vi "TrajectoryBegin.vi"(8 "error in (no error)":errorcluster) -> (0 "error out":errorcluster)   [LabVIEW 2023]
uses:
  TrajectoryGlobals.vi
  <vilib>/Rock Robotics/WPI/ThirdParty/JAS_Junk/TrajLib/Trajectory_Library.lvlib
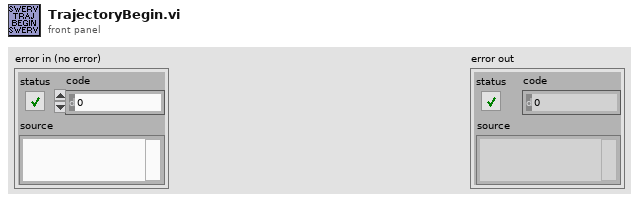
[diagram p1: front panel]
types:
  T1 = typedef "Trajectory_Library.lvlib/TRAJECTORY.ctl" = cluster{"TotalTImeSecs":dbl, "States":T2[]}
  T2 = typedef "Trajectory_Library.lvlib/TRAJ_STATE.ctl" = cluster{"TimeSeconds":dbl, "Velocity":dbl, "Acceleration":dbl, "POSE":T3, "Curvature":dbl}
  T3 = typedef "Trajectory_Library.lvlib/POSE2D.ctl" = cluster{"TRANSLATION":T4, "ROTATION":T5}
  T4 = typedef "Trajectory_Library.lvlib/TRANSLATION2D.ctl" = cluster{"X":dbl, "Y":dbl}
  T5 = typedef "Trajectory_Library.lvlib/ROTATION2D.ctl" = cluster{"VALUE":dbl, "COS":dbl, "SIN":dbl}
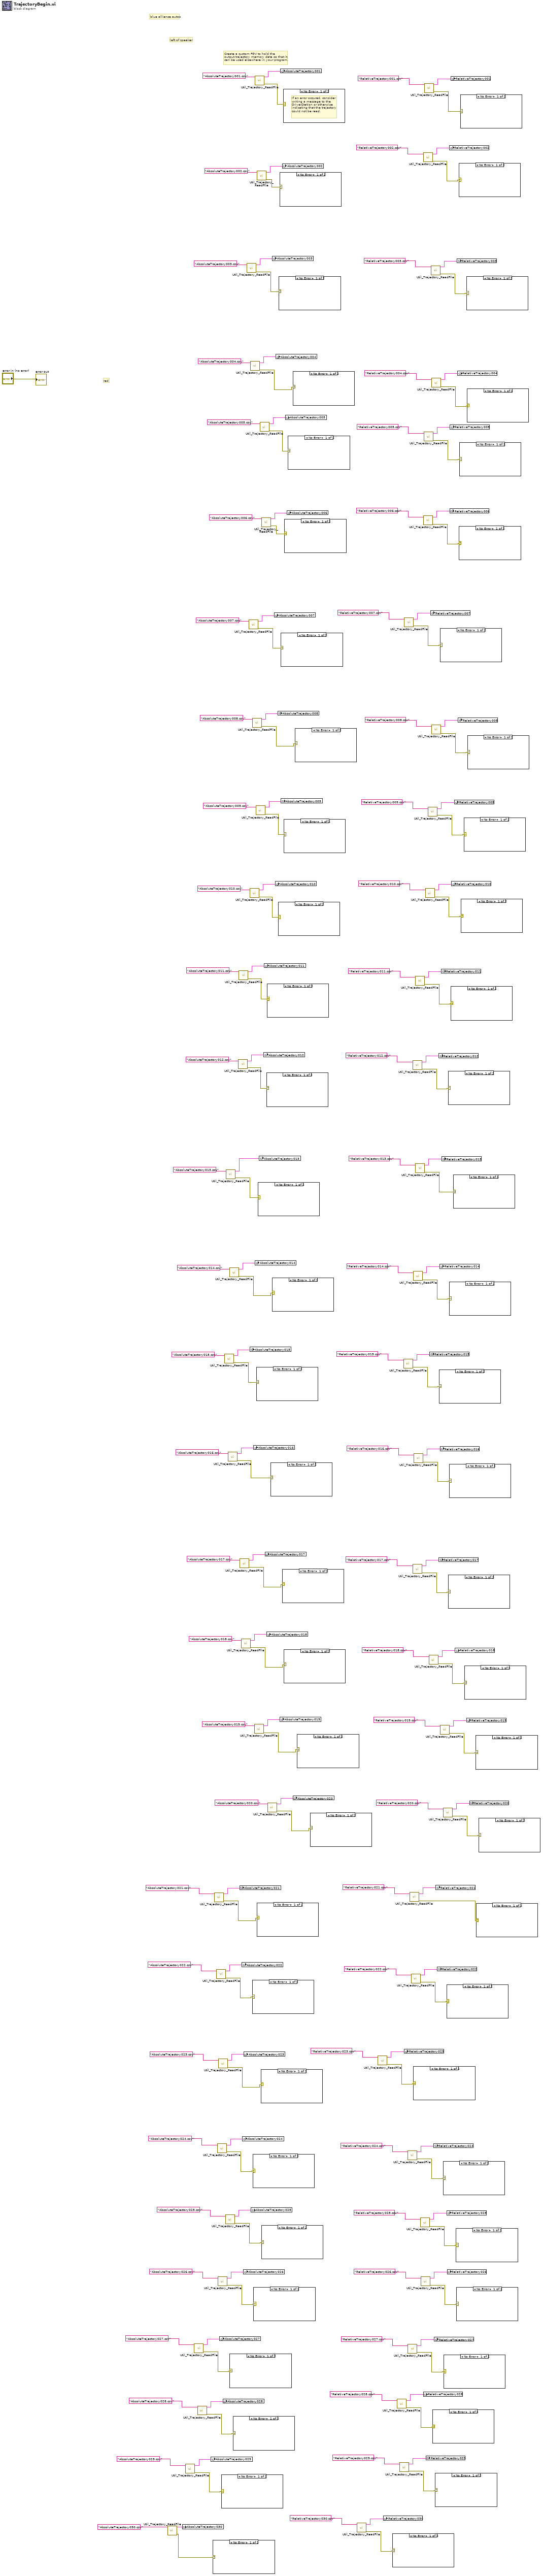
[diagram p0: block diagram]
diagram:
  # "red"
  # "Create a custom FGV to hold the \noutput trajectory memory data so that it\ncan be used elsewhere in your program."
  # "left of speaker"
  # "blue allience autos"
  n1 = call <vilib>:"Util_Trajectory_ReadFile.vi"("FileName"="AbsoluteTrajectory030.csv") -> ("error out"=w91:errorcluster, "outTRAJECTORY"=w92:T1)  [unwired: 8 in, 1 out]
  n2 = global write "TrajectoryGlobals.vi" "AbsoluteTrajectory030"(w92) -> ()
  n3 = call <vilib>:"Util_Trajectory_ReadFile.vi"("FileName"="AbsoluteTrajectory029.csv") -> ("error out"=w94:errorcluster, "outTRAJECTORY"=w95:T1)  [unwired: 8 in, 1 out]
  n4 = call <vilib>:"Util_Trajectory_ReadFile.vi"("FileName"="AbsoluteTrajectory027.csv") -> ("error out"=w100:errorcluster, "outTRAJECTORY"=w101:T1)  [unwired: 8 in, 1 out]
  n5 = call <vilib>:"Util_Trajectory_ReadFile.vi"("FileName"="AbsoluteTrajectory028.csv") -> ("error out"=w97:errorcluster, "outTRAJECTORY"=w98:T1)  [unwired: 8 in, 1 out]
  n6 = global write "TrajectoryGlobals.vi" "AbsoluteTrajectory029"(w95) -> ()
  n7 = case shown="No Error" w91 {
    frame No Error {
    }
    frame Error {
    }
  }
  n8 = call <vilib>:"Util_Trajectory_ReadFile.vi"("FileName"="AbsoluteTrajectory021.csv") -> ("error out"=w118:errorcluster, "outTRAJECTORY"=w119:T1)  [unwired: 8 in, 1 out]
  n9 = call <vilib>:"Util_Trajectory_ReadFile.vi"("FileName"="AbsoluteTrajectory022.csv") -> ("error out"=w115:errorcluster, "outTRAJECTORY"=w116:T1)  [unwired: 8 in, 1 out]
  n10 = call <vilib>:"Util_Trajectory_ReadFile.vi"("FileName"="AbsoluteTrajectory024.csv") -> ("error out"=w109:errorcluster, "outTRAJECTORY"=w110:T1)  [unwired: 8 in, 1 out]
  n11 = call <vilib>:"Util_Trajectory_ReadFile.vi"("FileName"="AbsoluteTrajectory026.csv") -> ("error out"=w103:errorcluster, "outTRAJECTORY"=w104:T1)  [unwired: 8 in, 1 out]
  n12 = call <vilib>:"Util_Trajectory_ReadFile.vi"("FileName"="AbsoluteTrajectory023.csv") -> ("error out"=w112:errorcluster, "outTRAJECTORY"=w113:T1)  [unwired: 8 in, 1 out]
  n13 = global write "TrajectoryGlobals.vi" "AbsoluteTrajectory027"(w101) -> ()
  n14 = case shown="No Error" w94 {
    frame No Error {
    }
    frame Error {
    }
  }
  n15 = global write "TrajectoryGlobals.vi" "AbsoluteTrajectory028"(w98) -> ()
  n16 = call <vilib>:"Util_Trajectory_ReadFile.vi"("FileName"="AbsoluteTrajectory015.csv") -> ("error out"=w142:errorcluster, "outTRAJECTORY"=w143:T1)  [unwired: 8 in, 1 out]
  n17 = call <vilib>:"Util_Trajectory_ReadFile.vi"("FileName"="AbsoluteTrajectory025.csv") -> ("error out"=w106:errorcluster, "outTRAJECTORY"=w107:T1)  [unwired: 8 in, 1 out]
  n18 = call <vilib>:"Util_Trajectory_ReadFile.vi"("FileName"="AbsoluteTrajectory013.csv") -> ("error out"=w136:errorcluster, "outTRAJECTORY"=w137:T1)  [unwired: 8 in, 1 out]
  n19 = call <vilib>:"Util_Trajectory_ReadFile.vi"("FileName"="AbsoluteTrajectory016.csv") -> ("error out"=w139:errorcluster, "outTRAJECTORY"=w140:T1)  [unwired: 8 in, 1 out]
  n20 = call <vilib>:"Util_Trajectory_ReadFile.vi"("FileName"="AbsoluteTrajectory014.csv") -> ("error out"=w133:errorcluster, "outTRAJECTORY"=w134:T1)  [unwired: 8 in, 1 out]
  n21 = case shown="No Error" w100 {
    frame No Error {
    }
    frame Error {
    }
  }
  n22 = case shown="No Error" w97 {
    frame No Error {
    }
    frame Error {
    }
  }
  n23 = call <vilib>:"Util_Trajectory_ReadFile.vi"("FileName"="AbsoluteTrajectory012.csv") -> ("error out"=w147:errorcluster, "outTRAJECTORY"=w145:T1)  [unwired: 8 in, 1 out]
  n24 = call <vilib>:"Util_Trajectory_ReadFile.vi"("FileName"="AbsoluteTrajectory011.csv") -> ("error out"=w150:errorcluster, "outTRAJECTORY"=w148:T1)  [unwired: 8 in, 1 out]
  n25 = call <vilib>:"Util_Trajectory_ReadFile.vi"("FileName"="AbsoluteTrajectory017.csv") -> ("error out"=w130:errorcluster, "outTRAJECTORY"=w131:T1)  [unwired: 8 in, 1 out]
  n26 = global write "TrajectoryGlobals.vi" "AbsoluteTrajectory021"(w119) -> ()
  n27 = call <vilib>:"Util_Trajectory_ReadFile.vi"("FileName"="AbsoluteTrajectory018.csv") -> ("error out"=w127:errorcluster, "outTRAJECTORY"=w128:T1)  [unwired: 8 in, 1 out]
  n28 = global write "TrajectoryGlobals.vi" "AbsoluteTrajectory022"(w116) -> ()
  n29 = global write "TrajectoryGlobals.vi" "AbsoluteTrajectory024"(w110) -> ()
  n30 = global write "TrajectoryGlobals.vi" "AbsoluteTrajectory026"(w104) -> ()
  n31 = global write "TrajectoryGlobals.vi" "AbsoluteTrajectory023"(w113) -> ()
  n32 = call <vilib>:"Util_Trajectory_ReadFile.vi"("FileName"="AbsoluteTrajectory003.csv") -> ("error out"=w160:errorcluster, "outTRAJECTORY"=w161:T1)  [unwired: 8 in, 1 out]
  n33 = call <vilib>:"Util_Trajectory_ReadFile.vi"("FileName"="AbsoluteTrajectory007.csv") -> ("error out"=w172:errorcluster, "outTRAJECTORY"=w173:T1)  [unwired: 8 in, 1 out]
  n34 = call <vilib>:"Util_Trajectory_ReadFile.vi"("FileName"="AbsoluteTrajectory010.csv") -> ("error out"=w153:errorcluster, "outTRAJECTORY"=w151:T1)  [unwired: 8 in, 1 out]
  n35 = global write "TrajectoryGlobals.vi" "AbsoluteTrajectory015"(w143) -> ()
  n36 = call <vilib>:"Util_Trajectory_ReadFile.vi"("FileName"="AbsoluteTrajectory004.csv") -> ("error out"=w157:errorcluster, "outTRAJECTORY"=w158:T1)  [unwired: 8 in, 1 out]
  n37 = global write "TrajectoryGlobals.vi" "AbsoluteTrajectory025"(w107) -> ()
  n38 = case shown="No Error" w115 {
    frame No Error {
    }
    frame Error {
    }
  }
  n39 = call <vilib>:"Util_Trajectory_ReadFile.vi"("FileName"="AbsoluteTrajectory008.csv") -> ("error out"=w169:errorcluster, "outTRAJECTORY"=w170:T1)  [unwired: 8 in, 1 out]
  n40 = case shown="No Error" w109 {
    frame No Error {
    }
    frame Error {
    }
  }
  n41 = global write "TrajectoryGlobals.vi" "AbsoluteTrajectory016"(w140) -> ()
  n42 = case shown="No Error" w103 {
    frame No Error {
    }
    frame Error {
    }
  }
  n43 = call <vilib>:"Util_Trajectory_ReadFile.vi"("FileName"="AbsoluteTrajectory019.csv") -> ("error out"=w124:errorcluster, "outTRAJECTORY"=w125:T1)  [unwired: 8 in, 1 out]
  n44 = global write "TrajectoryGlobals.vi" "AbsoluteTrajectory014"(w134) -> ()
  n45 = call <vilib>:"Util_Trajectory_ReadFile.vi"("FileName"="AbsoluteTrajectory001.csv") -> ("error out"=w168:errorcluster, "outTRAJECTORY"=w166:T1)  [unwired: 8 in, 1 out]
  n46 = call <vilib>:"Util_Trajectory_ReadFile.vi"("FileName"="AbsoluteTrajectory009.csv") -> ("error out"=w156:errorcluster, "outTRAJECTORY"=w154:T1)  [unwired: 8 in, 1 out]
  n47 = case shown="No Error" w142 {
    frame No Error {
    }
    frame Error {
    }
  }
  n48 = call <vilib>:"Util_Trajectory_ReadFile.vi"("FileName"="AbsoluteTrajectory002.csv") -> ("error out"=w163:errorcluster, "outTRAJECTORY"=w164:T1)  [unwired: 8 in, 1 out]
  n49 = case shown="No Error" w118 {
    frame No Error {
    }
    frame Error {
    }
  }
  n50 = case shown="No Error" w136 {
    frame No Error {
    }
    frame Error {
    }
  }
  n51 = global write "TrajectoryGlobals.vi" "AbsoluteTrajectory013"(w137) -> ()
  n52 = call <vilib>:"Util_Trajectory_ReadFile.vi"("FileName"="AbsoluteTrajectory005.csv") -> ("error out"=w180:errorcluster, "outTRAJECTORY"=w178:T1)  [unwired: 8 in, 1 out]
  n53 = case shown="No Error" w112 {
    frame No Error {
    }
    frame Error {
    }
  }
  n54 = case shown="No Error" w106 {
    frame No Error {
    }
    frame Error {
    }
  }
  n55 = call <vilib>:"Util_Trajectory_ReadFile.vi"("FileName"="AbsoluteTrajectory006.csv") -> ("error out"=w175:errorcluster, "outTRAJECTORY"=w176:T1)  [unwired: 8 in, 1 out]
  n56 = global write "TrajectoryGlobals.vi" "AbsoluteTrajectory012"(w145) -> ()
  n57 = global write "TrajectoryGlobals.vi" "AbsoluteTrajectory011"(w148) -> ()
  n58 = global write "TrajectoryGlobals.vi" "AbsoluteTrajectory017"(w131) -> ()
  n59 = case shown="No Error" w147 {
    frame No Error {
    }
    frame Error {
    }
  }
  n60 = global write "TrajectoryGlobals.vi" "AbsoluteTrajectory018"(w128) -> ()
  n61 = case shown="No Error" w150 {
    frame No Error {
    }
    frame Error {
    }
  }
  n62 = call <vilib>:"Util_Trajectory_ReadFile.vi"("FileName"="AbsoluteTrajectory020.csv") -> ("error out"=w121:errorcluster, "outTRAJECTORY"=w122:T1)  [unwired: 8 in, 1 out]
  n63 = case shown="No Error" w139 {
    frame No Error {
    }
    frame Error {
    }
  }
  n64 = global write "TrajectoryGlobals.vi" "AbsoluteTrajectory003"(w161) -> ()
  n65 = case shown="No Error" w133 {
    frame No Error {
    }
    frame Error {
    }
  }
  n66 = global write "TrajectoryGlobals.vi" "AbsoluteTrajectory007"(w173) -> ()
  n67 = global write "TrajectoryGlobals.vi" "AbsoluteTrajectory010"(w151) -> ()
  n68 = global write "TrajectoryGlobals.vi" "AbsoluteTrajectory004"(w158) -> ()
  n69 = global write "TrajectoryGlobals.vi" "AbsoluteTrajectory008"(w170) -> ()
  n70 = case shown="No Error" w153 {
    frame No Error {
    }
    frame Error {
    }
  }
  n71 = case shown="No Error" w160 {
    frame No Error {
    }
    frame Error {
    }
  }
  n72 = case shown="No Error" w163 {
    frame No Error {
    }
    frame Error {
    }
  }
  n73 = global write "TrajectoryGlobals.vi" "AbsoluteTrajectory019"(w125) -> ()
  n74 = global write "TrajectoryGlobals.vi" "AbsoluteTrajectory001"(w166) -> ()
  n75 = case shown="No Error" w172 {
    frame No Error {
    }
    frame Error {
    }
  }
  n76 = global write "TrajectoryGlobals.vi" "AbsoluteTrajectory009"(w154) -> ()
  n77 = global write "TrajectoryGlobals.vi" "AbsoluteTrajectory002"(w164) -> ()
  n78 = case shown="No Error" w130 {
    frame No Error {
    }
    frame Error {
    }
  }
  n79 = case shown="No Error" w168 {
    frame No Error {
      # "If an error occured, consider\nwriting a message to the\nDriverStation or otherwise\nindicating that the trajectory\ncould not be read."
    }
    frame Error {
    }
  }
  n80 = case shown="No Error" w156 {
    frame No Error {
    }
    frame Error {
    }
  }
  n81 = case shown="No Error" w127 {
    frame No Error {
    }
    frame Error {
    }
  }
  n82 = case shown="No Error" w175 {
    frame No Error {
    }
    frame Error {
    }
  }
  n83 = global write "TrajectoryGlobals.vi" "AbsoluteTrajectory005"(w178) -> ()
  n84 = global write "TrajectoryGlobals.vi" "AbsoluteTrajectory006"(w176) -> ()
  n85 = case shown="No Error" w180 {
    frame No Error {
    }
    frame Error {
    }
  }
  n86 = global write "TrajectoryGlobals.vi" "AbsoluteTrajectory020"(w122) -> ()
  n87 = case shown="No Error" w157 {
    frame No Error {
    }
    frame Error {
    }
  }
  n88 = case shown="No Error" w169 {
    frame No Error {
    }
    frame Error {
    }
  }
  n89 = case shown="No Error" w124 {
    frame No Error {
    }
    frame Error {
    }
  }
  n90 = case shown="No Error" w121 {
    frame No Error {
    }
    frame Error {
    }
  }
  n91 = call <vilib>:"Util_Trajectory_ReadFile.vi"("FileName"="RelativeTrajectory030.csv") -> ("error out"=w1:errorcluster, "outTRAJECTORY"=w2:T1)  [unwired: 8 in, 1 out]
  n92 = call <vilib>:"Util_Trajectory_ReadFile.vi"("FileName"="RelativeTrajectory023.csv") -> ("error out"=w22:errorcluster, "outTRAJECTORY"=w23:T1)  [unwired: 8 in, 1 out]
  n93 = global write "TrajectoryGlobals.vi" "RelativeTrajectory030"(w2) -> ()
  n94 = case shown="No Error" w1 {
    frame No Error {
    }
    frame Error {
    }
  }
  n95 = call <vilib>:"Util_Trajectory_ReadFile.vi"("FileName"="RelativeTrajectory028.csv") -> ("error out"=w7:errorcluster, "outTRAJECTORY"=w8:T1)  [unwired: 8 in, 1 out]
  n96 = call <vilib>:"Util_Trajectory_ReadFile.vi"("FileName"="RelativeTrajectory029.csv") -> ("error out"=w4:errorcluster, "outTRAJECTORY"=w5:T1)  [unwired: 8 in, 1 out]
  n97 = call <vilib>:"Util_Trajectory_ReadFile.vi"("FileName"="RelativeTrajectory015.csv") -> ("error out"=w46:errorcluster, "outTRAJECTORY"=w47:T1)  [unwired: 8 in, 1 out]
  n98 = global write "TrajectoryGlobals.vi" "RelativeTrajectory023"(w23) -> ()
  n99 = call <vilib>:"Util_Trajectory_ReadFile.vi"("FileName"="RelativeTrajectory007.csv") -> ("error out"=w70:errorcluster, "outTRAJECTORY"=w71:T1)  [unwired: 8 in, 1 out]
  n100 = call <vilib>:"Util_Trajectory_ReadFile.vi"("FileName"="RelativeTrajectory024.csv") -> ("error out"=w19:errorcluster, "outTRAJECTORY"=w20:T1)  [unwired: 8 in, 1 out]
  n101 = call <vilib>:"Util_Trajectory_ReadFile.vi"("FileName"="RelativeTrajectory027.csv") -> ("error out"=w10:errorcluster, "outTRAJECTORY"=w11:T1)  [unwired: 8 in, 1 out]
  n102 = call <vilib>:"Util_Trajectory_ReadFile.vi"("FileName"="RelativeTrajectory021.csv") -> ("error out"=w28:errorcluster, "outTRAJECTORY"=w29:T1)  [unwired: 8 in, 1 out]
  n103 = call <vilib>:"Util_Trajectory_ReadFile.vi"("FileName"="RelativeTrajectory022.csv") -> ("error out"=w25:errorcluster, "outTRAJECTORY"=w26:T1)  [unwired: 8 in, 1 out]
  n104 = call <vilib>:"Util_Trajectory_ReadFile.vi"("FileName"="RelativeTrajectory012.csv") -> ("error out"=w55:errorcluster, "outTRAJECTORY"=w56:T1)  [unwired: 8 in, 1 out]
  n105 = call <vilib>:"Util_Trajectory_ReadFile.vi"("FileName"="RelativeTrajectory017.csv") -> ("error out"=w40:errorcluster, "outTRAJECTORY"=w41:T1)  [unwired: 8 in, 1 out]
  n106 = call <vilib>:"Util_Trajectory_ReadFile.vi"("FileName"="RelativeTrajectory014.csv") -> ("error out"=w49:errorcluster, "outTRAJECTORY"=w50:T1)  [unwired: 8 in, 1 out]
  n107 = case shown="No Error" w22 {
    frame No Error {
    }
    frame Error {
    }
  }
  n108 = call <vilib>:"Util_Trajectory_ReadFile.vi"("FileName"="RelativeTrajectory016.csv") -> ("error out"=w43:errorcluster, "outTRAJECTORY"=w44:T1)  [unwired: 8 in, 1 out]
  n109 = call <vilib>:"Util_Trajectory_ReadFile.vi"("FileName"="RelativeTrajectory011.csv") -> ("error out"=w58:errorcluster, "outTRAJECTORY"=w59:T1)  [unwired: 8 in, 1 out]
  n110 = call <vilib>:"Util_Trajectory_ReadFile.vi"("FileName"="RelativeTrajectory013.csv") -> ("error out"=w52:errorcluster, "outTRAJECTORY"=w53:T1)  [unwired: 8 in, 1 out]
  n111 = call <vilib>:"Util_Trajectory_ReadFile.vi"("FileName"="RelativeTrajectory025.csv") -> ("error out"=w16:errorcluster, "outTRAJECTORY"=w17:T1)  [unwired: 8 in, 1 out]
  n112 = call <vilib>:"Util_Trajectory_ReadFile.vi"("FileName"="RelativeTrajectory026.csv") -> ("error out"=w13:errorcluster, "outTRAJECTORY"=w14:T1)  [unwired: 8 in, 1 out]
  n113 = call <vilib>:"Util_Trajectory_ReadFile.vi"("FileName"="RelativeTrajectory002.csv") -> ("error out"=w85:errorcluster, "outTRAJECTORY"=w86:T1)  [unwired: 8 in, 1 out]
  n114 = global write "TrajectoryGlobals.vi" "RelativeTrajectory028"(w8) -> ()
  n115 = call <vilib>:"Util_Trajectory_ReadFile.vi"("FileName"="RelativeTrajectory006.csv") -> ("error out"=w73:errorcluster, "outTRAJECTORY"=w74:T1)  [unwired: 8 in, 1 out]
  n116 = call <vilib>:"Util_Trajectory_ReadFile.vi"("FileName"="RelativeTrajectory005.csv") -> ("error out"=w76:errorcluster, "outTRAJECTORY"=w77:T1)  [unwired: 8 in, 1 out]
  n117 = call <vilib>:"Util_Trajectory_ReadFile.vi"("FileName"="RelativeTrajectory001.csv") -> ("error out"=w88:errorcluster, "outTRAJECTORY"=w89:T1)  [unwired: 8 in, 1 out]
  n118 = call <vilib>:"Util_Trajectory_ReadFile.vi"("FileName"="RelativeTrajectory010.csv") -> ("error out"=w61:errorcluster, "outTRAJECTORY"=w62:T1)  [unwired: 8 in, 1 out]
  n119 = global write "TrajectoryGlobals.vi" "RelativeTrajectory029"(w5) -> ()
  n120 = call <vilib>:"Util_Trajectory_ReadFile.vi"("FileName"="RelativeTrajectory009.csv") -> ("error out"=w64:errorcluster, "outTRAJECTORY"=w65:T1)  [unwired: 8 in, 1 out]
  n121 = call <vilib>:"Util_Trajectory_ReadFile.vi"("FileName"="RelativeTrajectory018.csv") -> ("error out"=w34:errorcluster, "outTRAJECTORY"=w35:T1)  [unwired: 8 in, 1 out]
  n122 = global write "TrajectoryGlobals.vi" "RelativeTrajectory015"(w47) -> ()
  n123 = global write "TrajectoryGlobals.vi" "RelativeTrajectory007"(w71) -> ()
  n124 = call <vilib>:"Util_Trajectory_ReadFile.vi"("FileName"="RelativeTrajectory003.csv") -> ("error out"=w82:errorcluster, "outTRAJECTORY"=w83:T1)  [unwired: 8 in, 1 out]
  n125 = call <vilib>:"Util_Trajectory_ReadFile.vi"("FileName"="RelativeTrajectory004.csv") -> ("error out"=w79:errorcluster, "outTRAJECTORY"=w80:T1)  [unwired: 8 in, 1 out]
  n126 = call <vilib>:"Util_Trajectory_ReadFile.vi"("FileName"="RelativeTrajectory008.csv") -> ("error out"=w67:errorcluster, "outTRAJECTORY"=w68:T1)  [unwired: 8 in, 1 out]
  n127 = case shown="No Error" w7 {
    frame No Error {
    }
    frame Error {
    }
  }
  n128 = global write "TrajectoryGlobals.vi" "RelativeTrajectory024"(w20) -> ()
  n129 = global write "TrajectoryGlobals.vi" "RelativeTrajectory027"(w11) -> ()
  n130 = case shown="No Error" w4 {
    frame No Error {
    }
    frame Error {
    }
  }
  n131 = global write "TrajectoryGlobals.vi" "RelativeTrajectory021"(w29) -> ()
  n132 = global write "TrajectoryGlobals.vi" "RelativeTrajectory022"(w26) -> ()
  n133 = global write "TrajectoryGlobals.vi" "RelativeTrajectory012"(w56) -> ()
  n134 = global write "TrajectoryGlobals.vi" "RelativeTrajectory017"(w41) -> ()
  n135 = case shown="No Error" w46 {
    frame No Error {
    }
    frame Error {
    }
  }
  n136 = global write "TrajectoryGlobals.vi" "RelativeTrajectory014"(w50) -> ()
  n137 = case shown="No Error" w70 {
    frame No Error {
    }
    frame Error {
    }
  }
  n138 = global write "TrajectoryGlobals.vi" "RelativeTrajectory016"(w44) -> ()
  n139 = call <vilib>:"Util_Trajectory_ReadFile.vi"("FileName"="RelativeTrajectory019.csv") -> ("error out"=w37:errorcluster, "outTRAJECTORY"=w38:T1)  [unwired: 8 in, 1 out]
  n140 = global write "TrajectoryGlobals.vi" "RelativeTrajectory011"(w59) -> ()
  n141 = global write "TrajectoryGlobals.vi" "RelativeTrajectory013"(w53) -> ()
  n142 = call <vilib>:"Util_Trajectory_ReadFile.vi"("FileName"="RelativeTrajectory020.csv") -> ("error out"=w31:errorcluster, "outTRAJECTORY"=w32:T1)  [unwired: 8 in, 1 out]
  n143 = case shown="No Error" w19 {
    frame No Error {
    }
    frame Error {
    }
  }
  n144 = case shown="No Error" w10 {
    frame No Error {
    }
    frame Error {
    }
  }
  n145 = case shown="No Error" w25 {
    frame No Error {
    }
    frame Error {
    }
  }
  n146 = global write "TrajectoryGlobals.vi" "RelativeTrajectory025"(w17) -> ()
  n147 = global write "TrajectoryGlobals.vi" "RelativeTrajectory026"(w14) -> ()
  n148 = case shown="No Error" w55 {
    frame No Error {
    }
    frame Error {
    }
  }
  n149 = case shown="No Error" w40 {
    frame No Error {
    }
    frame Error {
    }
  }
  n150 = case shown="No Error" w49 {
    frame No Error {
    }
    frame Error {
    }
  }
  n151 = global write "TrajectoryGlobals.vi" "RelativeTrajectory002"(w86) -> ()
  n152 = case shown="No Error" w43 {
    frame No Error {
    }
    frame Error {
    }
  }
  n153 = global write "TrajectoryGlobals.vi" "RelativeTrajectory006"(w74) -> ()
  n154 = global write "TrajectoryGlobals.vi" "RelativeTrajectory005"(w77) -> ()
  n155 = global write "TrajectoryGlobals.vi" "RelativeTrajectory001"(w89) -> ()
  n156 = case shown="No Error" w58 {
    frame No Error {
    }
    frame Error {
    }
  }
  n157 = global write "TrajectoryGlobals.vi" "RelativeTrajectory010"(w62) -> ()
  n158 = case shown="No Error" w52 {
    frame No Error {
    }
    frame Error {
    }
  }
  n159 = global write "TrajectoryGlobals.vi" "RelativeTrajectory009"(w65) -> ()
  n160 = global write "TrajectoryGlobals.vi" "RelativeTrajectory018"(w35) -> ()
  n161 = case shown="No Error" w16 {
    frame No Error {
    }
    frame Error {
    }
  }
  n162 = case shown="No Error" w13 {
    frame No Error {
    }
    frame Error {
    }
  }
  n163 = global write "TrajectoryGlobals.vi" "RelativeTrajectory003"(w83) -> ()
  n164 = global write "TrajectoryGlobals.vi" "RelativeTrajectory004"(w80) -> ()
  n165 = global write "TrajectoryGlobals.vi" "RelativeTrajectory008"(w68) -> ()
  n166 = case shown="No Error" w85 {
    frame No Error {
    }
    frame Error {
    }
  }
  n167 = case shown="No Error" w73 {
    frame No Error {
    }
    frame Error {
    }
  }
  n168 = case shown="No Error" w76 {
    frame No Error {
    }
    frame Error {
    }
  }
  n169 = case shown="No Error" w88 {
    frame No Error {
    }
    frame Error {
    }
  }
  n170 = case shown="No Error" w61 {
    frame No Error {
    }
    frame Error {
    }
  }
  n171 = case shown="No Error" w64 {
    frame No Error {
    }
    frame Error {
    }
  }
  n172 = case shown="No Error" w34 {
    frame No Error {
    }
    frame Error {
    }
  }
  n173 = case shown="No Error" w82 {
    frame No Error {
    }
    frame Error {
    }
  }
  n174 = global write "TrajectoryGlobals.vi" "RelativeTrajectory019"(w38) -> ()
  n175 = case shown="No Error" w79 {
    frame No Error {
    }
    frame Error {
    }
  }
  n176 = case shown="No Error" w67 {
    frame No Error {
    }
    frame Error {
    }
  }
  n177 = global write "TrajectoryGlobals.vi" "RelativeTrajectory020"(w32) -> ()
  n178 = case shown="No Error" w37 {
    frame No Error {
    }
    frame Error {
    }
  }
  n179 = case shown="No Error" w28 {
    frame No Error {
    }
    frame Error {
    }
  }
  n180 = case shown="No Error" w31 {
    frame No Error {
    }
    frame Error {
    }
  }
  "error out" <- "error in (no error)"
